vi "TPIStageInit.vi"(1 "error in (no error)":errorcluster) -> (0 "error out":errorcluster)   [LabVIEW 2009]
uses:
  StageSettings.ctt
  <vilib>/Utility/config.llb/NI_LVConfig.lvlib
panel:
  out "PI Stage Setup":T1={"channels (x, y, z)"="2", "Stage Scaling (V/µm)"=0.1} {"Stage Scaling (V/µm)" format="%.2f"}
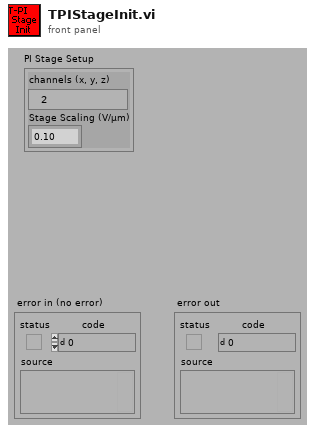
[diagram p1: front panel]
types:
  T1 = typedef "StageSettings.ctt" = cluster{"channels (x, y, z)":tag, "Stage Scaling (V/µm)":dbl}
  T2 = typedef "NI_LVConfig.lvlib/Config Data RefNum.ctl" = refnum<k1>
  T3 = cluster{"channels (x, y, z)":tag, "Stage Scaling (V/µm)":dbl}
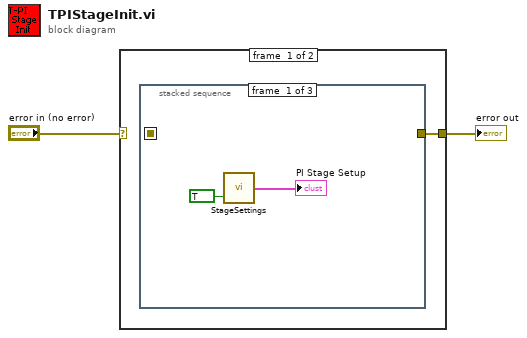
[diagram p0: block diagram]
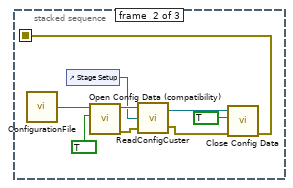
[diagram p2: hidden frame]
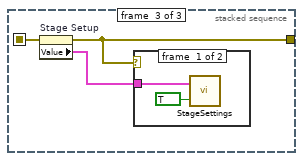
[diagram p3: hidden frame]
diagram:
  n1 = case shown="No Error" "error in (no error)" {
    selector: "error in (no error)" -> [_ w20]
    tunnel: [w3 w20] -> w1
    frame #0 {
      n2 = stacked-sequence {
        seq-local: [_ w10 _] -> [_ _ w17]
        tunnel: [_ _ w16] -> w3
        frame #0 {
          n3 = call "StageSettings.vi"("Get/Set"=TRUE) -> ("PI Stage Setup (output)"=→"PI Stage Setup":T1)  [unwired: 1 in]
        }
        frame #1 {
          n4 = call "ConfigurationFile.vi"() -> ("Configuration File (output)"=w9:path)  [unwired: 2 in]
          n5 = control-ref of="Stage Setup"() -> (w8:refnum<vi>)
          n6 = call <vilib>:"Open Config Data (compatibility).vi"("create file if necessary (T)"=TRUE ("create file if necessary? (T)"), "configuration file path"=w9) -> ("error out"=w12:errorcluster, "refnum"=w13:T2)  [unwired: 7 in, 1 out]
          n7 = call "ReadConfigCuster.vi"("error in (no error)"=w12, "Ctrl Reference"=w8, "ConfigFile (input)"=w13) -> ("error out"=w6:errorcluster, "ConfigFile (output)"=w7:T2)
          n8 = call "Close Config Data.vi"("error in (no error)"=w6, "write configuration file? (T)"=TRUE ("write configuration file? (F)"), "refnum"=w7) -> ("error out"=w10:errorcluster)  [unwired: 8 in]
        }
        frame #2 {
          n9 = property on="Stage Setup" class="Clust (strict)"(error in=w17) -> (error out=w16:errorcluster, "Value"=w15:T3)  [unwired: 1 in, 1 out]
          n10 = case shown="No Error" w16 {
            tunnel: w15 -> [w18 _]
            frame #0 {
              n11 = call "StageSettings.vi"("Get/Set"=TRUE ("Set"), "PI Stage Setup (input)"=w18) -> ()  [unwired: 1 out]
            }
            frame #1 {
            }
          }
        }
      }
    }
    frame #1 {
    }
  }
  "error out" <- w1
